vi "28_March_lite.vi"() -> ()   [LabVIEW 2021]
uses:
  <vilib>/Platform/TimedLoop/XDataNode/timing_clust.ctl
  <vilib>/Platform/TimedLoop/XDataNode/nitl_modes.ctl
  <vilib>/Platform/TimedLoop/XDataNode/wakeup.ctl
  <vilib>/Analysis/2dsp.llb/Real FFT.vi
  <vilib>/Analysis/5stat.llb/RMS (DBL).vi
  <vilib>/Utility/file.llb/Write Delimited Spreadsheet (DBL).vi
  <vilib>/Platform/TimedLoop/XDataNode/loadnilvce.vi
  <vilib>/FPGAPlugInAG/cRIO-9045/niLvFpga_Open_cRIO-9045.vi
  <vilib>/rvi/interface/common/dynamic/niFpgaDynamicAddResources.vi
  <vilib>/rvi/interface/common/niFpgaWaitOnOcc.vi
  <vilib>/Utility/error.llb/Error Cluster From Error Code.vi
  <vilib>/rvi/errors/niLvFpgaAdjustHostInterfaceError.vi
  <vilib>/FPGAPlugInAG/Dynamic/niLvFpga_Close_Dynamic.vi
  <vilib>/platform/TimedLoop/XDataNode/XDataNode.xnode
  <vilib>/rvi/interface/nirviOpenFPGA/nirviOpenFPGA.xnode
  D:/KHANH/FPGA Bitfiles/labviewbaitap_FPGATarget_FPGAtest_zBSNpXufBbI.lvbitx
  D:/KHANH/FPGA_test.vi
  <vilib>/rvi/interface/nirviMethod/nirviMethod.xnode
  <vilib>/rvi/interface/nirviReadWriteControl/nirviReadWriteControl.xnode
  <vilib>/rvi/interface/nirviCloseFPGA/nirviCloseFPGA.xnode
  <vilib>/Platform/TimedLoop/XDataNode/XDNodeRunTimeDep.lvlib
  <vilib>/Analysis/NI_AALPro.lvlib
  <vilib>/rvi/errors/niLvFpgaMergeErrorWithErrorCode.vi
  <vilib>/FPGAPlugInAG/Dynamic/niLvFpga_ConfigureFifo_Dynamic.vi
  NiFpgaLv.dll
  <vilib>/rvi/interface/Simulation/niFpgaSimulationCallBeginRW.vi
  <vilib>/FPGAPlugInAG/Dynamic/niLvFpga_ReadFifo_Dynamic.vi
panel:
  out "unsigned 8bit integer":u8
  out "Boolean 2":bool
  out "Numeric":sgl
  out "Row":string[](array[string])=["Channel 1  ", "Channel 2 ", "Channel 3 "]
  in  "Main tab":enum32{"Intro", "Control", "Simulation"}(tab)
  out "RMS Vel.":dbl
  out "Boolean":bool
  in  "Reset Button":bool
  in  "Measure Button":bool
  out "Max Disp 3":dbl
  out "Max Disp 2":dbl
  out "Max Disp":dbl
  out "RMS Vel.":dbl
  out "RMS Vel.":dbl
  out "real_meas_time":dbl
  in  "Measurement time (s)":dbl=1.0 min=0.0 max=1500.0
  in  "Sampling frequency (Hz)":dbl max=10000.0 step=1000.0
  in  "Frequency \nresolution deltaF":dbl step=0.1
  in  "Start Button":bool
  in  "Tab Control 2":T1(tab)
  out "Channel 1 Displacement":dbl[](graph)
  out "FFT channel 1":cluster{i32, dbl, dbl[]}(graph)
  out "Channel 2 Data":sgl[](graph)
  out "FFT channel 2":cluster{i32, dbl, dbl[]}(graph)
  out "Channel 3 Data":sgl[](graph)
  out "FFT channel 3":cluster{i32, dbl, dbl[]}(graph)
  in  "Tab Control":enum32{"Measurement", "Recording"}(tab)
  out "Current Value":string[][](array[string])
  out "Measurement result":string[][](array[string])
  in  "Number of cycle":dbl
  out "Over Threshold ?":bool
  in  "Specify Threshold":dbl=4.5 min=4.5 max=10.0 step=1.0
  out "Number of reading buffer  2":u32
  in  "buffer size":i32
  out "buffer for 1 channel":dbl
  out "recording buffer":dbl[](array[numeric])
  in  "Number of reading buffer":u32
  out "to PC overflow?":bool
  out "Samples remaining":u32
  out "Actual Depth":u32
  out "Acceleration\nPosition 2":dbl
  out "Acceleration\nPosition 1":dbl
  in  "stop":bool
  out "Date & Time":string
  out "Disp.":dbl[](array[numeric])
  out "Disp.":sgl[](array[numeric])
  out "Disp.":sgl[](array[numeric])
  in  "stop 2":bool
  in  "DIRECTION ON/OFF":bool
  in  "PWM0":dbl(slide) caption="PWM0 (% Duty Cycle)" scale=0.0..100.0
  in  "PWM1":dbl(slide) caption="PWM1 (% Duty Cycle)" scale=0.0..100.0
  in  "Stop":bool
  out "String":string="Loi deltaF = 0"
  out "shared channel":sgl[][](array[numeric])
  out "channel 1":sgl[](array[numeric])
  # "CAPSTONE PROJECT"
  # "REAL-TIME VIBRATION MONITORING SYSTEM"
  # "CVT REAL-TIME VIBRATION MONITORING SYSTEM"
  # "Control"
  # "Configurations"
  # "Measurement"
  # "deltaF = Fs / N \nfs = sampling frequency \nN = number of samples"
  # "Piezoelectric Icp Accelerometer 333B40"
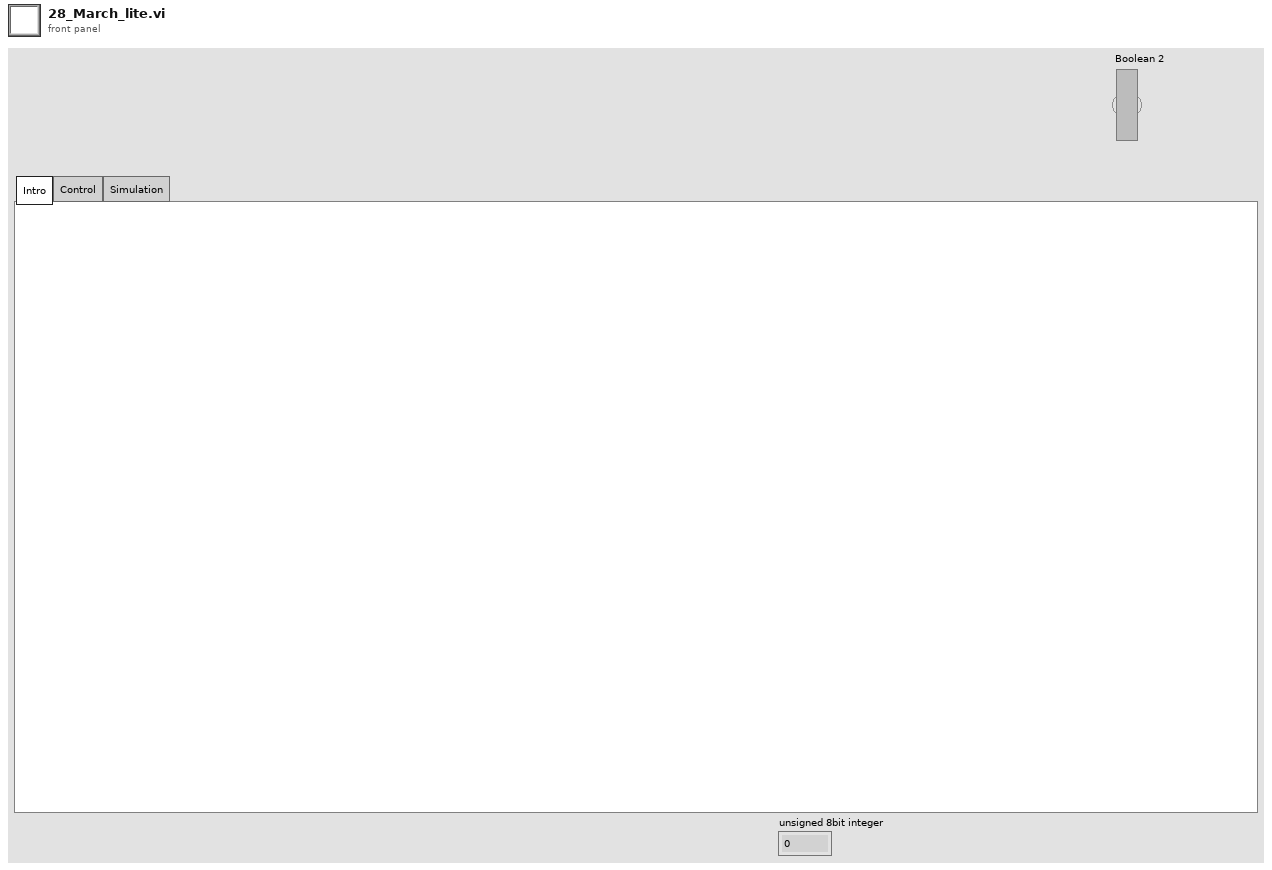
[diagram p1: front panel]
types:
  T1 = enum32{"Channel 1  ", "Channel 2", "Channel 3 ", "Measurement", "Service", "BeltBox"}
  T2 = typedef "XDNodeRunTimeDep.lvlib/timing_clust.ctl" = cluster{"Expected End [f-1]":u64, "Actual End [f-1]":u64, "Finished Late? [f-1]":bool, "Expected End [i-1]":u64, "Actual End [i-1]":u64, "Finished Late? [i-1]":bool, "Expected Start [i]":u64, "Actual Start [i]":u64, "Expected Start [f]":u64, "Actual Start [f]":u64, "Source Name":string, "Structure Name":string, "Period":i64, "Deadline":i64, "Offset":i64, "Start":i64, "Priority":i32, "Timeout":i32, "Mode":T3, "Wakeup Reason":T4, "Error":errorcluster, "Source Type":string, "Secondary Source Type":string, "Global End Time":u64, "Global Start Time":u64, "Frame Duration":u64, "Iteration Duration":u64, "Assigned CPU":i32, "I/O Scan Engine Mode":u32}
  T3 = typedef "XDNodeRunTimeDep.lvlib/nitl_modes.ctl" = enum32{"No Change", "Process missed periods, maintain original phase", "Discard missed periods, maintain original phase", "Process missed periods, ignore original phase", "Discard missed periods, ignore original phase"}
  T4 = typedef "XDNodeRunTimeDep.lvlib/wakeup.ctl" = enum32{"Normal", "Aborted", "Asynchronous wakeup", "Timing source error", "Timed loop error", "Timeout"}
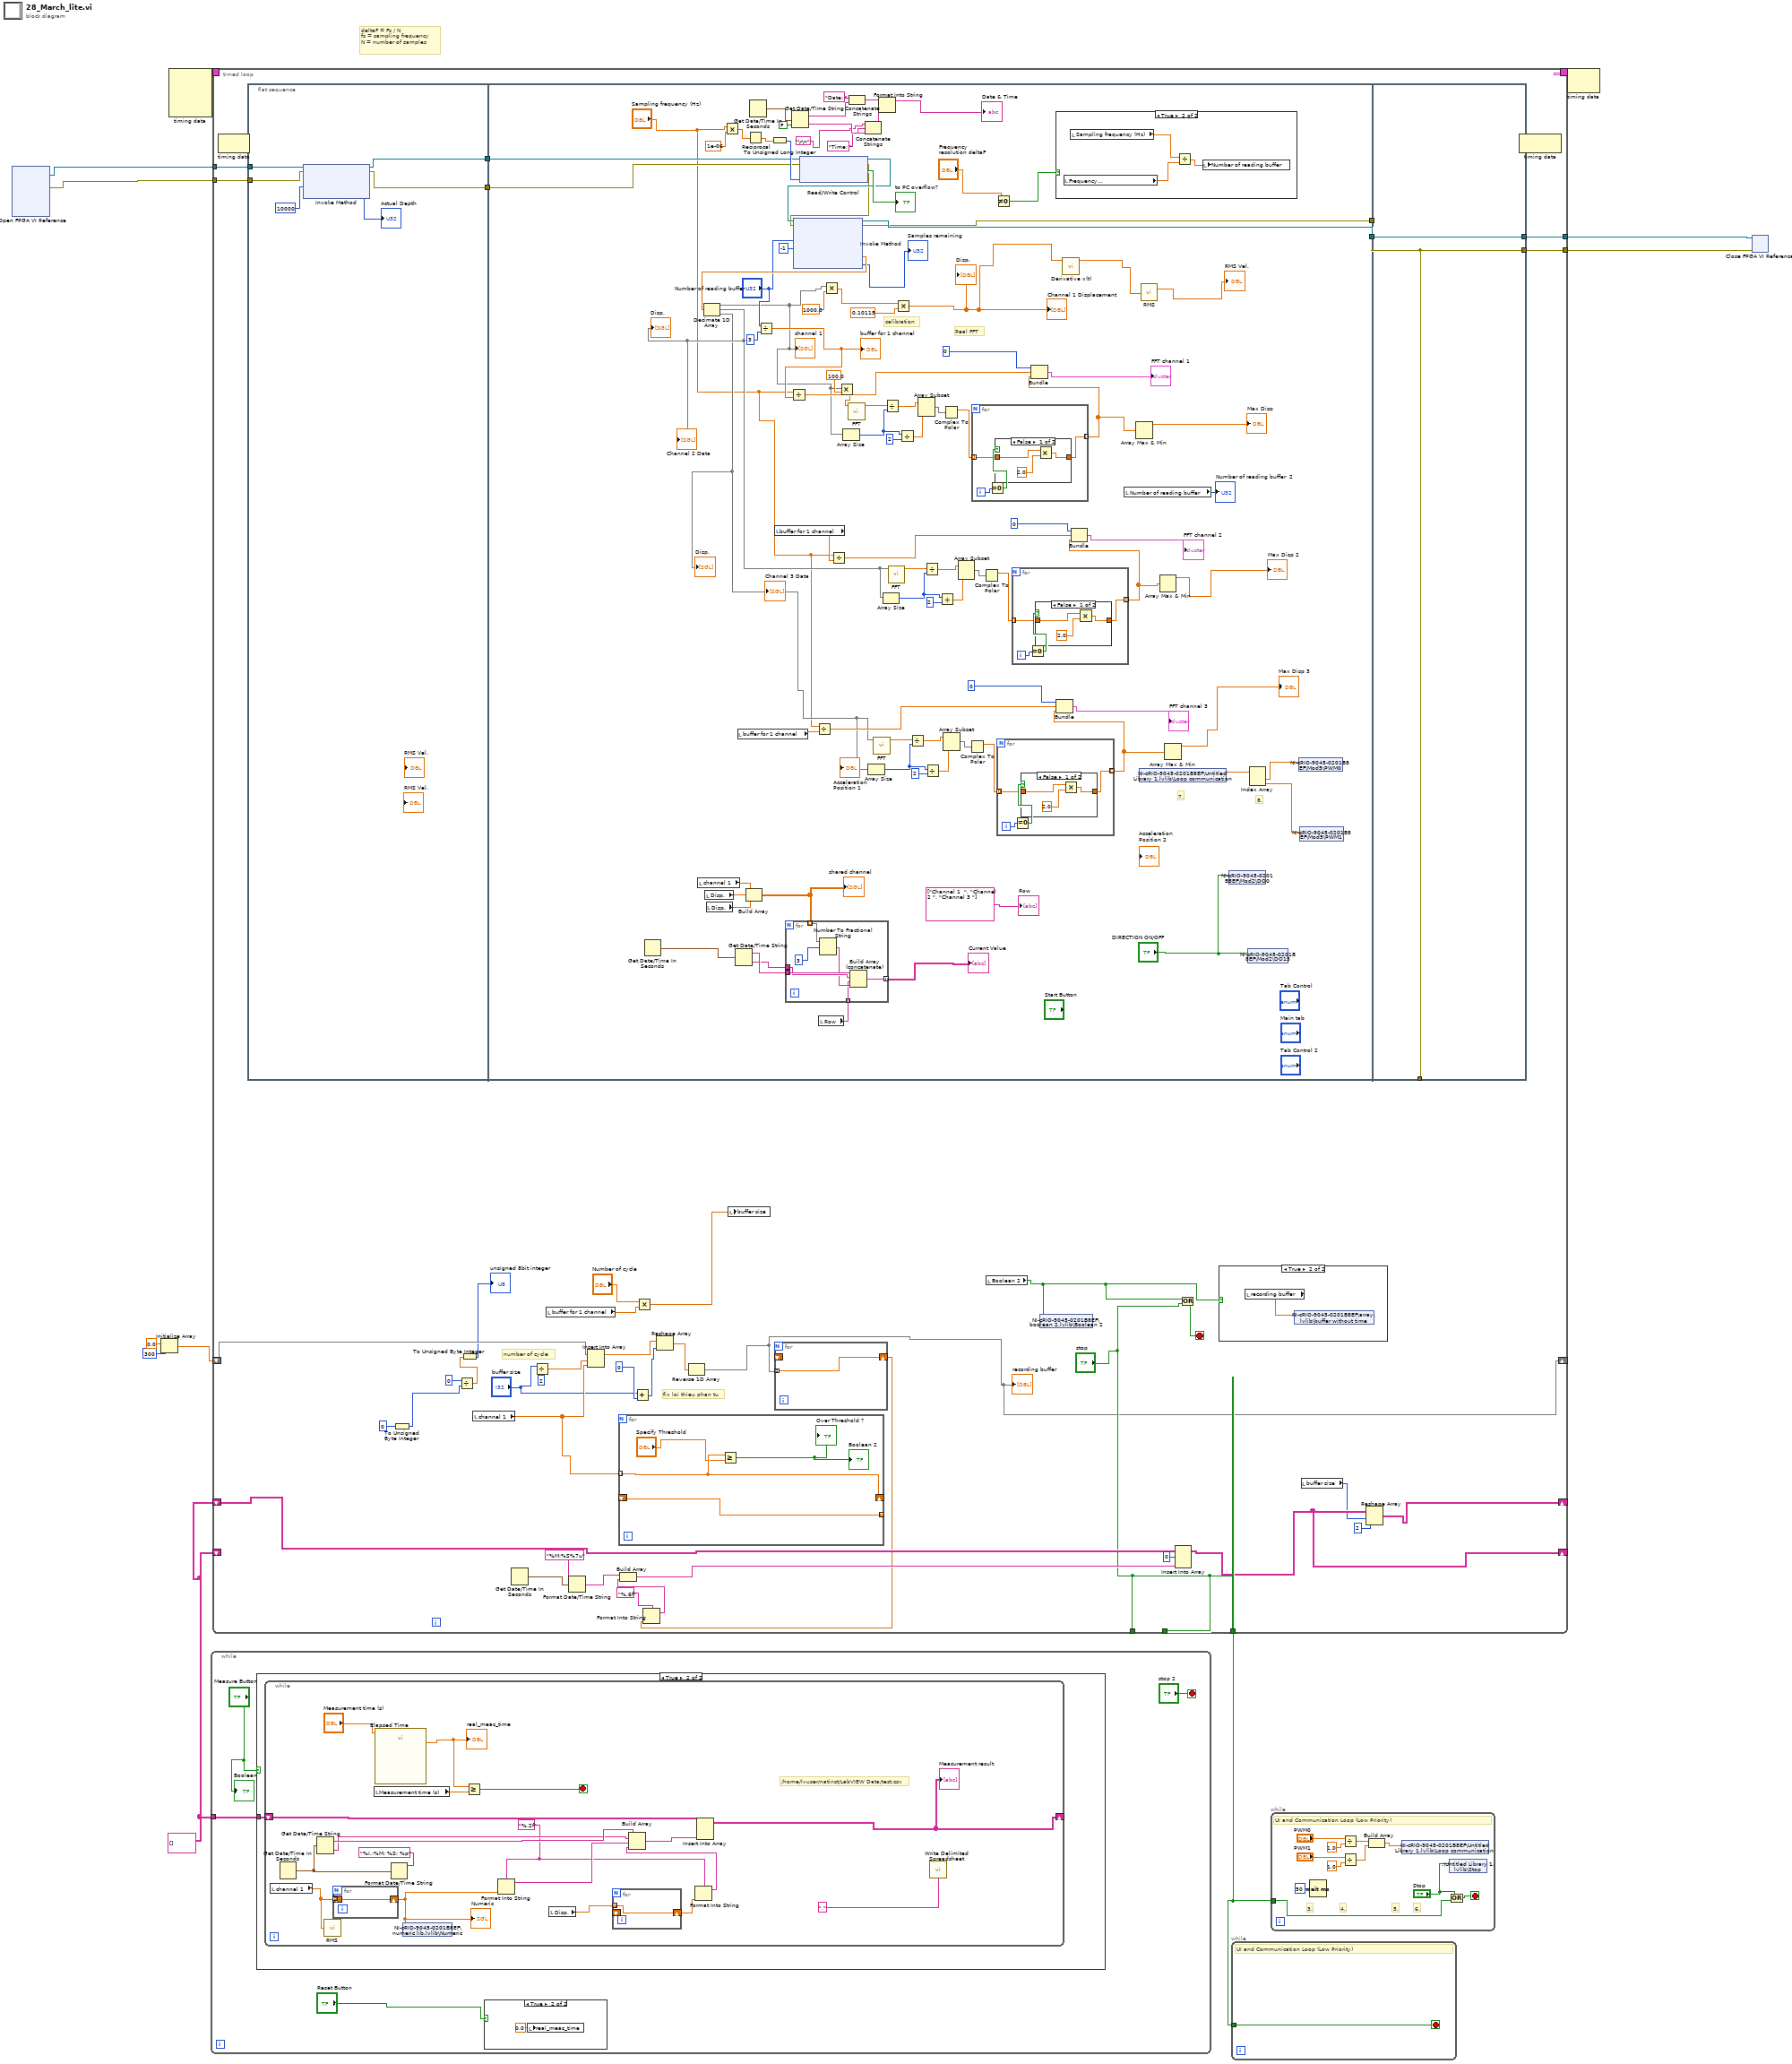
[diagram p0: block diagram]
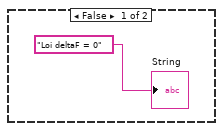
[diagram p5: hidden frame]
diagram:
  w5 = string[][] []
  # "deltaF = Fs / N \nfs = sampling frequency \nN = number of samples"
  n1 = xnode "Open FPGA VI Reference"() -> ("FPGA VI Reference Out"=w7:refnum<k20>, "error out"=w6:errorcluster)  [unwired: 2 in]
  n2 = Initialize Array(0.0 ("element"), 300 ("dimension size")) -> (w3:dbl[])
  n3 = node-c288() -> (w11:T2)  [unwired: 4 in]
  n4 = while {
    tunnel: w5 -> [w15]
    stop <- "stop 2" stop-if-true
    n5 = case shown="True" "Measure Button" {
      tunnel: w15 -> [_ w17]
      frame False {
      }
      frame True {
        n6 = while {
          shift-right: [w25] -> _
          shift-left: w17 -> [w27]
          stop <- w33 stop-if-true
          w19 = "%.2f" ("format string")
          # "/home/lvuser/natinst/LabVIEW Data/test.csv"
          n7 = local read "channel 1"() -> (w22:sgl[])
          n8 = Get Date/Time In Seconds() -> (seconds since 1Jan1904=w32:timestamp)
          n9 = Get Date/Time String(seconds (now)=w32) -> (date string=w31:string, time string=w26:string)  [unwired: 2 in]
          n10 = call-poly <vilib>:"RMS.vi"("X"=w22) -> ()  [unwired: 2 out]
          n11 = for {
            tunnel: w22 -> [w38] mode=indexing
            shift-right: [w38] -> w23
            shift-left: _ -> [_]
          }
          "Numeric" <- w23
          n12 = local read "Measurement time (s)"() -> (w34:dbl)
          n13 = call "Elapsed Time"("Time Target (s)"="Measurement time (s)") -> ("Elapsed Time (s)"=w35:dbl)  [unwired: 11 in, 7 out]
          "real_meas_time" <- w35
          n14 = Format Date/Time String(time format string (%c)="%I,;%M; %S; %p", seconds (now)=w32) -> ()  [unwired: 1 in, 1 out]
          n15 = shared-variable "NI-cRIO-9045-0201B8EF\\numeric lib.lvlib\\Numeric"(w23) -> ()  [unwired: 1 in, 1 out]
          n16 = Greater Or Equal?(x=w35, y=w34) -> (x >= y?=w33:bool)
          n17 = Format Into String(format string=w19, w23) -> (resulting string=w30:string)  [unwired: 2 in, 1 out]
          n18 = local read "Disp."() -> (w21:sgl[])
          n19 = for {
            tunnel: w21 -> [w37] mode=indexing
            shift-right: [w37] -> w20
            shift-left: _ -> [_]
          }
          n20 = Format Into String(format string=w19, w20) -> (resulting string=w18:string)  [unwired: 2 in, 1 out]
          n21 = Build Array(w31, w26, w30, w18) -> (w29:string[])
          n22 = Insert Into Array(array=w27, new element=w29) -> (w25:string[][])  [unwired: 2 in]
          "Measurement result" <- w25
          n23 = call-poly <vilib>:"Write Delimited Spreadsheet.vi"("delimiter (\\t)"="," ("delimiter (\\t)")) -> ()  [unwired: 13 in, 2 out]
        }
      }
    }
    n24 = case shown="True" "Reset Button" {
      frame False {
      }
      frame True {
        n25 = local write "real_meas_time"(0.0 ("real_meas_time")) -> ()
      }
    }
    "Boolean" <- "Measure Button"
  }
  n26 = timed-loop {
    timing: w11 -> [_]
    timing-out: [_] -> w10
    tunnel: ["stop"] -> w4
    tunnel: [w76] -> w9
    tunnel: [w75] -> w8
    shift-right: [w51] -> _
    shift-left: w3 -> [w54]
    tunnel: ["stop"] -> _
    tunnel: w7 -> [w74]
    tunnel: w6 -> [w73]
    shift-right: [w66] -> _
    shift-left: w5 -> [_]
    shift-right: [w65] -> _
    shift-left: w5 -> [w64]
    tunnel: ["stop"] -> _
    stop <- w61 stop-if-true
    # "number of cycle"
    # "fix loi thieu phan tu"
    n27 = node-c288() -> ()  [unwired: 1 in, 1 out]
    n28 = flat-sequence {
      tunnel: [w89] -> w78
      tunnel: [w90] -> w77
      tunnel: w74 -> [w92]
      tunnel: w73 -> [w91]
      tunnel: [w186] -> w80
      tunnel: [w185] -> w79
      tunnel: w78 -> [w125]
      tunnel: w77 -> [w124]
      tunnel: w80 -> [w223]
      tunnel: w79 -> [w222]
      tunnel: [w222] -> _
      tunnel: [w223] -> w76
      tunnel: [w222] -> w75
      frame #0 {
        n29 = xnode "Invoke Method"("FPGA VI Reference In"=w92, "error in"=w91, "Requested Depth"=u32 10000) -> ("FPGA VI Reference Out"=w89:refnum<k20>, "error out"=w90:errorcluster, "Actual Depth"=→"Actual Depth":u32)
      }
      frame #1 {
        # "calibration"
        # "8."
        # "7."
        # "Real FFT"
        n30 = Get Date/Time In Seconds() -> (seconds since 1Jan1904=w100:timestamp)
        n31 = local read "channel 1"() -> (w117:sgl[])
        n32 = local read "Disp."() -> (w127:sgl[])
        n33 = local read "Disp."() -> (w126:sgl[])
        n34 = Multiply(x="Sampling frequency (Hz)", y=1e-06) -> (x*y=w164:dbl)
        n35 = Get Date/Time String(seconds (now)=w100) -> (date string=w181:string, time string=w180:string)  [unwired: 2 in]
        n36 = local read "buffer for 1 channel"() -> (w135:dbl)
        n37 = Build Array(w117, w127, w126) -> (w182:sgl[][])
        "shared channel" <- w182
        n38 = Reciprocal(x=w164) -> (1/x=w163:dbl)
        n39 = Get Date/Time In Seconds() -> (seconds since 1Jan1904=w112:timestamp)
        n40 = Divide(x="Number of reading buffer", y=u32 3) -> (x/y=w137:dbl)
        "buffer for 1 channel" <- w137
        n41 = To Unsigned Long Integer(number=w163) -> (unsigned 32bit integer=w167:u32)
        n42 = local read "buffer for 1 channel"() -> (w136:dbl)
        n43 = Divide(x="Sampling frequency (Hz)", y=w137) -> (x/y=w178:dbl)
        n44 = Get Date/Time String(seconds (now)=w112, want seconds? (F)=FALSE) -> (date string=w108:string, time string=w106:string)  [unwired: 1 in]
        n45 = xnode "Read/Write Control"("FPGA VI Reference In"=w125, "error in"=w124, "Sampling frequency"=w167) -> ("FPGA VI Reference Out"=w169:refnum<k20>, "error out"=w168:errorcluster, "Timed Out? 2"=→"to PC overflow?":bool)
        n46 = xnode "Invoke Method"("FPGA VI Reference In"=w169, "error in"=w168, "Number of Elements"="Number of reading buffer", "Timeout (ms)"=-1) -> ("FPGA VI Reference Out"=w186:refnum<k20>, "error out"=w185:errorcluster, "Data"=w162:sgl[], "Elements Remaining"=→"Samples remaining":u32)
        n47 = Decimate 1D Array(w162) -> (w103:sgl[], w142:sgl[], w140:sgl[])
        "channel 1" <- w103
        "Channel 2 Data" <- w142
        "Channel 3 Data" <- w140
        "Disp." <- w142
        "Disp." <- w140
        n48 = Divide(x="Sampling frequency (Hz)", y=w135) -> (x/y=w151:dbl)
        n49 = local read "Row"() -> (w122:string[])
        n50 = for {
          tunnel: w182 -> [w221] mode=indexing
          tunnel: w181 -> [w219]
          tunnel: w180 -> [w218]
          tunnel: [w216] -> w118 mode=indexing
          tunnel: w122 -> [w215] mode=indexing
          n51 = Number To Fractional String(number=w221, width (-)=i16 3) -> (F-format string=w217:string[])  [unwired: 2 in]
          n52 = Build Array (concatenate)(w219, w218, w215, w217) -> (w216:string[])
        }
        "Current Value" <- w118
        n53 = Multiply(x=w103, y=1000.0) -> (x*y=w101:dbl[])
        n54 = Divide(x="Sampling frequency (Hz)", y=w136) -> (x/y=w160:dbl)
        n55 = Multiply(x=w103, y=100.0) -> (x*y=w133:dbl[])
        n56 = Array Size(array=w103) -> (size(s)=w175:i32)
        n57 = call-poly <vilib>:"FFT.vi"("X"=w133) -> ("FFT {X}"=w179:cdb[])  [unwired: 9 in, 1 out]
        n58 = Concatenate Strings("Date: ", w108) -> (w109:string)
        n59 = Concatenate Strings("\r\n", "Time: ", w106) -> (w110:string)
        n60 = Array Size(array=w140) -> (size(s)=w149:i32)
        n61 = call-poly <vilib>:"FFT.vi"("X"=w140) -> ("FFT {X}"=w152:cdb[])  [unwired: 9 in, 1 out]
        n62 = Format Into String(initial string=w109, w110) -> (resulting string=→"Date & Time":string)  [unwired: 2 in, 1 out]
        n63 = Array Size(array=w142) -> (size(s)=w158:i32)
        n64 = Divide(x=w179, y=w175) -> (x/y=w172:cdb[])
        n65 = call-poly <vilib>:"FFT.vi"("X"=w142) -> ("FFT {X}"=w161:cdb[])  [unwired: 9 in, 1 out]
        n66 = Multiply(x=w101, y=0.10115) -> (x*y=w95:dbl[])
        "Channel 1 Displacement" <- w95
        "Disp." <- w95
        n67 = Divide(x=w175, y=2) -> (x/y=w173:dbl)
        n68 = Divide(x=w152, y=w149) -> (x/y=w146:cdb[])
        n69 = Array Subset(array=w172, length=w173) -> (w171:cdb[])  [unwired: 1 in]
        n70 = Divide(x=w161, y=w158) -> (x/y=w155:cdb[])
        n71 = Divide(x=w149, y=2) -> (x/y=w147:dbl)
        n72 = Divide(x=w158, y=2) -> (x/y=w156:dbl)
        n73 = Complex To Polar(r * e^(i*theta)=w171) -> (r=w170:dbl[])  [unwired: 1 out]
        n74 = Array Subset(array=w146, length=w147) -> (w145:cdb[])  [unwired: 1 in]
        n75 = Array Subset(array=w155, length=w156) -> (w154:cdb[])  [unwired: 1 in]
        n76 = Complex To Polar(r * e^(i*theta)=w145) -> (r=w144:dbl[])  [unwired: 1 out]
        n77 = for {
          tunnel: w170 -> [w208] mode=indexing
          tunnel: [w207] -> w116 mode=indexing
          i -> [w210]
          n78 = Equal To 0?(x=w210) -> (x = 0?=w209:bool)
          n79 = case shown="False" w209 {
            tunnel: [w211 w214] -> w207
            tunnel: w208 -> [w213 w214]
            frame False {
              n80 = Multiply(x=w213, y=2.0) -> (x*y=w211:dbl)
            }
            frame True {
            }
          }
        }
        n81 = Complex To Polar(r * e^(i*theta)=w154) -> (r=w153:dbl[])  [unwired: 1 out]
        n82 = Not Equal To 0?(x="Frequency \nresolution deltaF") -> (x != 0?=w99:bool)
        n83 = for {
          tunnel: w144 -> [w192] mode=indexing
          tunnel: [w191] -> w114 mode=indexing
          i -> [w194]
          n84 = Equal To 0?(x=w194) -> (x = 0?=w193:bool)
          n85 = case shown="False" w193 {
            tunnel: [w195 w198] -> w191
            tunnel: w192 -> [w197 w198]
            frame False {
              n86 = Multiply(x=w197, y=2.0) -> (x*y=w195:dbl)
            }
            frame True {
            }
          }
        }
        n87 = for {
          tunnel: w153 -> [w200] mode=indexing
          tunnel: [w199] -> w115 mode=indexing
          i -> [w202]
          n88 = Equal To 0?(x=w202) -> (x = 0?=w201:bool)
          n89 = case shown="False" w201 {
            tunnel: [w203 w206] -> w199
            tunnel: w200 -> [w205 w206]
            frame False {
              n90 = Multiply(x=w205, y=2.0) -> (x*y=w203:dbl)
            }
            frame True {
            }
          }
        }
        n91 = Bundle(0, w178, w116) -> (→"FFT channel 1":cluster{i32, dbl, dbl[]})  [unwired: 1 in]
        n92 = case shown="True" w99 {
          frame False {
            "String" <- "Loi deltaF = 0"
          }
          frame True {
            n93 = local read "Frequency \nresolution deltaF"() -> (w189:dbl)
            n94 = local read "Sampling frequency (Hz)"() -> (w190:dbl)
            n95 = Divide(x=w190, y=w189) -> (x/y=w188:dbl)
            n96 = local write "Number of reading buffer"(w188) -> ()
          }
        }
        n97 = Bundle(0, w151, w114) -> (→"FFT channel 3":cluster{i32, dbl, dbl[]})  [unwired: 1 in]
        n98 = call <vilib>:"Derivative x(t).vi"("X"=w95) -> ("dX/dt"=w94:dbl[])  [unwired: 9 in, 1 out]
        n99 = Bundle(0, w160, w115) -> (→"FFT channel 2":cluster{i32, dbl, dbl[]})  [unwired: 1 in]
        n100 = local read "Number of reading buffer"() -> (→"Number of reading buffer  2":u32)
        n101 = Array Max & Min(array=w116) -> (max value=→"Max Disp":dbl)  [unwired: 3 out]
        n102 = shared-variable "NI-cRIO-9045-0201B8EF\\Untitled Library 1.lvlib\\Loop communication"() -> (w132:dbl[])  [unwired: 1 in, 1 out]
        n103 = call-poly <vilib>:"RMS.vi"("X"=w94) -> ("rms value"=→"RMS Vel.":dbl)  [unwired: 1 out]
        n104 = Array Max & Min(array=w115) -> (max value=→"Max Disp 2":dbl)  [unwired: 3 out]
        n105 = Array Max & Min(array=w114) -> (max value=→"Max Disp 3":dbl)  [unwired: 3 out]
        n106 = shared-variable "NI-cRIO-9045-0201B8EF\\Mod2\\DO0"("DIRECTION ON/OFF") -> ()  [unwired: 1 in, 1 out]
        n107 = shared-variable "NI-cRIO-9045-0201B8EF\\Mod2\\DO15"("DIRECTION ON/OFF") -> ()  [unwired: 1 in, 1 out]
        n108 = Index Array(array=w132) -> (element #1=w131:dbl, element #2=w130:dbl)  [unwired: 2 in]
        n109 = shared-variable "NI-cRIO-9045-0201B8EF\\Mod5\\PWM0"(w131) -> ()  [unwired: 1 in, 1 out]
        n110 = shared-variable "NI-cRIO-9045-0201B8EF\\Mod5\\PWM1"(w130) -> ()  [unwired: 1 in, 1 out]
        "Row" <- string[] ["Channel 1  ", "Channel 2 ", "Channel 3 "]
      }
      frame #2 {
      }
    }
    n111 = To Unsigned Byte Integer(number=u8 0) -> (unsigned 8bit integer=w49:u8)
    n112 = Divide(x=u8 0, y=w49) -> (x/y=w47:dbl)
    n113 = To Unsigned Byte Integer(number=w47) -> (unsigned 8bit integer=→"unsigned 8bit integer":u8)
    n114 = local read "channel 1"() -> (w57:sgl[])
    n115 = Get Date/Time In Seconds() -> (seconds since 1Jan1904=w70:timestamp)
    n116 = Divide(x="buffer size", y=2) -> (x/y=w39:dbl)
    n117 = local read "buffer for 1 channel"() -> (w44:dbl)
    n118 = Format Date/Time String(time format string (%c)="%M:%S%7u", seconds (now)=w70) -> (date/time string=w58:string)  [unwired: 1 in]
    n119 = Insert Into Array "Insert Into Array"(array=w54, index=w39, new element=w57) -> (w56:dbl[])
    n120 = for {
      tunnel: w57 -> [w85] mode=indexing
      shift-right: [w85] -> _
      shift-left: _ -> [w86]
      tunnel: [w86] -> _ mode=indexing
      n121 = Greater Or Equal?(x=w85, y="Specify Threshold") -> (x >= y?=→"Over Threshold ?" →"Boolean 2":bool)
    }
    n122 = Add(x="buffer size", y=0) -> (x+y=w55:i32)
    n123 = Multiply(x="Number of cycle", y=w44) -> (x*y=w40:dbl)
    n124 = Reshape Array "Reshape Array"(w56, w55) -> (w53:dbl[])
    n125 = Reverse 1D Array(array=w53) -> (reversed array=w51:dbl[])
    "recording buffer" <- w51
    n126 = local write "buffer size"(w40) -> ()
    n127 = for {
      tunnel: w51 -> [w82] mode=indexing
      shift-right: [w82] -> w59
      shift-left: _ -> [_]
    }
    n128 = Format Into String(format string="%.6f", w59) -> (resulting string=w60:string)  [unwired: 2 in, 1 out]
    n129 = Build Array(w58, w60) -> (w68:string[])
    n130 = local read "Boolean 2"() -> (w50:bool)
    n131 = shared-variable "NI-cRIO-9045-0201B8EF\\boolean 2.lvlib\\Boolean 2"(w50) -> ()  [unwired: 1 in, 1 out]
    n132 = Insert Into Array(array=w64, index (row)=0, new element=w68) -> (w66:string[][])  [unwired: 1 in]
    n133 = Or(x=w50, y="stop") -> (x .or. y?=w61:bool)
    n134 = case shown="True" w50 {
      frame False {
      }
      frame True {
        n135 = local read "recording buffer"() -> (w81:dbl[])
        n136 = shared-variable "NI-cRIO-9045-0201B8EF\\array.lvlib\\buffer without time"(w81) -> ()  [unwired: 1 in, 1 out]
      }
    }
    n137 = local read "buffer size"() -> (w62:i32)
    n138 = Reshape Array(w66, w62, 2 ("dimension size")) -> (w65:string[][])
    n139 = node-c288() -> ()  [unwired: 1 in, 1 out]
  }
  n140 = while "UI and Communication Loop (Low Priority)" {
    tunnel: w4 -> [w226]
    stop <- w226 stop-if-true
    # "UI and Communication Loop (Low Priority)"
  }
  n141 = while "UI and Communication Loop (Low Priority)" {
    tunnel: w4 -> [w228]
    stop <- w227 stop-if-true
    # "3."
    # "5."
    # "4."
    # "6."
    # "UI and Communication Loop (Low Priority)"
    n142 = Wait (ms)(milliseconds to wait=u32 50 ("millisecond multiple")) -> ()  [unwired: 1 out]
    n143 = Divide(x="PWM0", y=1.0) -> (x/y=w236:dbl)
    n144 = Divide(x="PWM1", y=1.0) -> (x/y=w231:dbl)
    n145 = Build Array(w236, w231) -> (w230:dbl[])
    n146 = shared-variable "NI-cRIO-9045-0201B8EF\\Untitled Library 1.lvlib\\Loop communication"(w230) -> ()  [unwired: 1 in, 1 out]
    n147 = Or(x="Stop", y=w228) -> (x .or. y?=w227:bool)
    n148 = shared-variable ".\\Untitled Library 1.lvlib\\Stop"("Stop") -> ()  [unwired: 1 in, 1 out]
  }
  n149 = node-c288(w10) -> ()  [unwired: 1 out]
  n150 = xnode "Close FPGA VI Reference"("FPGA VI Reference In"=w9, "error in"=w8) -> ()  [unwired: 1 out]
